vi "Single_ASIC_L1_R_W.vi"(0 "connection ID":refnum<k5>, 1 "Register or channel":i32=96, 2 "RD/#WR":bool, 3 "error in (no error)":errorcluster, 4 "Data":u32) -> (5 "data out serial":string="0_2-63@36\r\n", 6 "connection ID out":refnum<k5>, 7 "data read value":u32=36, 9 "error out":errorcluster)   [LabVIEW 2012]
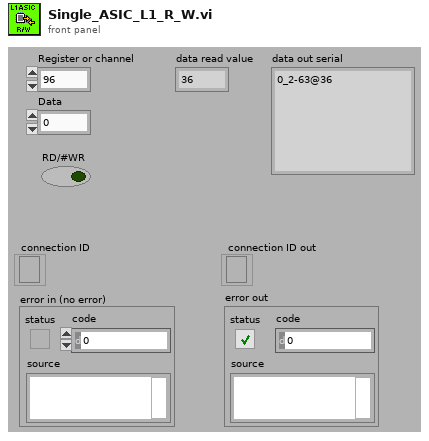
[diagram p1: front panel]
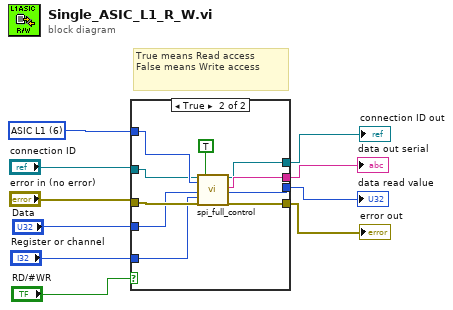
[diagram p0: block diagram]
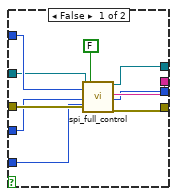
[diagram p2: hidden frame]
diagram:
  w5 = u16 6 items=["Attenuation", "Clipping", "Enable channel", "Delay line", "ASIC", "Enable L1 ch", "ASIC L1"] ("Device")
  # "True means Read access\nFalse means Write access"
  n1 = case shown="True" "RD/#WR" {
    tunnel: [w13 w29] -> w10
    tunnel: [w14 w28] -> w9
    tunnel: [w15 w27] -> w8
    tunnel: [w12 w26] -> w1
    tunnel: w5 -> [w19 w25]
    tunnel: "error in (no error)" -> [w17 w24]
    tunnel: "connection ID" -> [w18 w23]
    tunnel: "Register or channel" -> [w16 w22]
    tunnel: "Data" -> [w11 w21]
    frame False {
      n2 = call "spi_full_control.vi"("connection ID"=w18, "Device"=w19, "Data"=w11, "Register or channel"=w16, "error out 3"=w17, "Read physical"=FALSE) -> ("connection ID out"=w15:refnum<k5>, "data out serial"=w14:string, "data read value"=w13:u32, "error out 2"=w12:errorcluster)  [unwired: 6 in, 4 out]
    }
    frame True {
      n3 = call "spi_full_control.vi"("connection ID"=w23, "Device"=w25, "Data"=w21, "Register or channel"=w22, "error out 3"=w24, "Read physical"=TRUE) -> ("connection ID out"=w27:refnum<k5>, "data out serial"=w28:string, "data read value"=w29:u32, "error out 2"=w26:errorcluster)  [unwired: 6 in, 4 out]
    }
  }
  "data read value" <- w10
  "data out serial" <- w9
  "connection ID out" <- w8
  "error out" <- w1
